vi "methane_reactor_run.vi"() -> ()   [LabVIEW 2019]
uses:
  <vilib>/Utility/sysdir.llb/System Directory Type.ctl
  lib/libSimulationControl/libSimulationControl.lvlib
  lib/libFileFunctions/libFileFunctions.lvlib
panel:
  out "working_directory_tmp":string
  out "working_directory":string
  out "time":dbl
  out "starttime":dbl
  out "standard output":string
  out "standard error":string
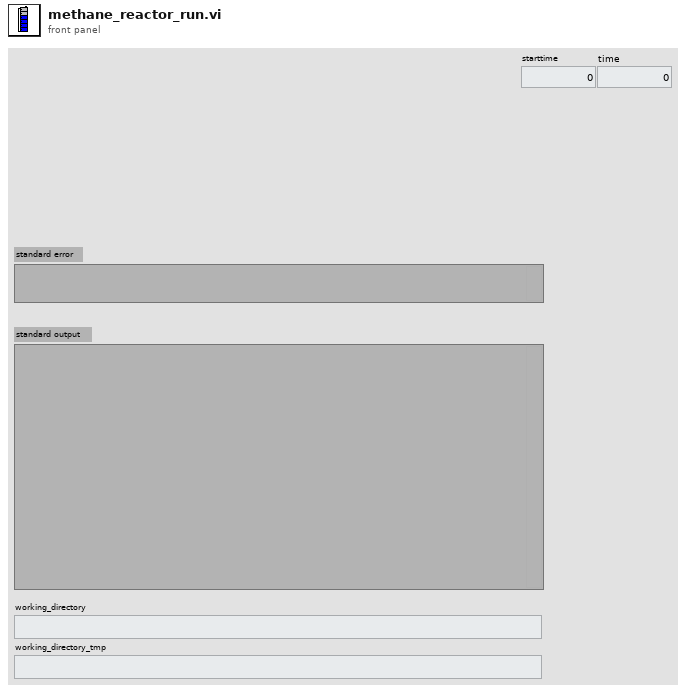
[diagram p1: front panel]
types:
  T1 = typedef "System Directory Type.ctl" = i32
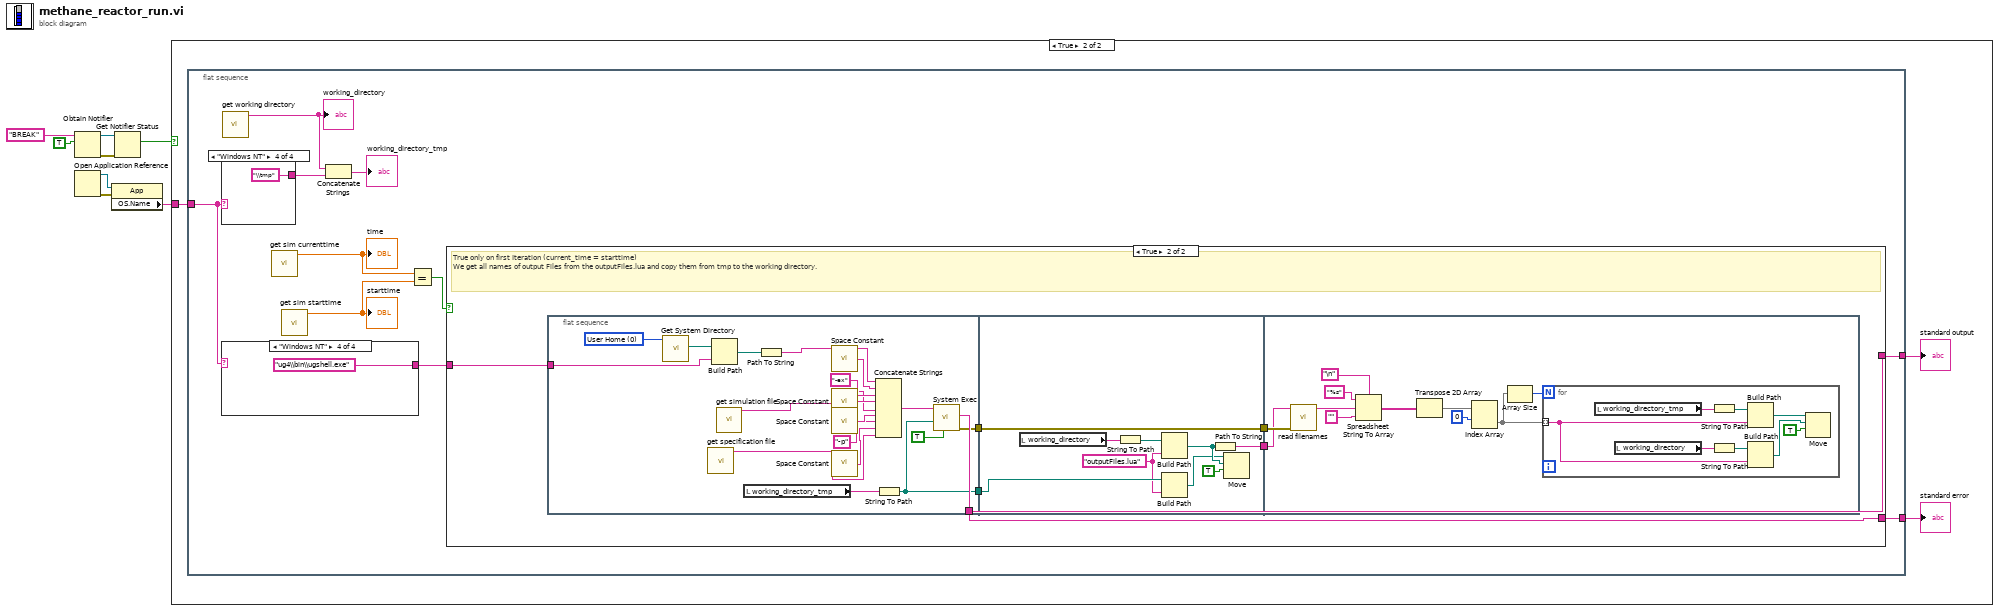
[diagram p0: block diagram]
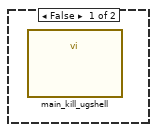
[diagram p2: hidden frame]
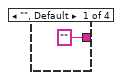
[diagram p3: hidden frame]
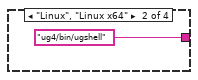
[diagram p4: hidden frame]
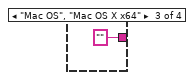
[diagram p5: hidden frame]
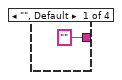
[diagram p6: hidden frame]
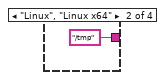
[diagram p7: hidden frame]
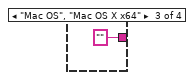
[diagram p8: hidden frame]
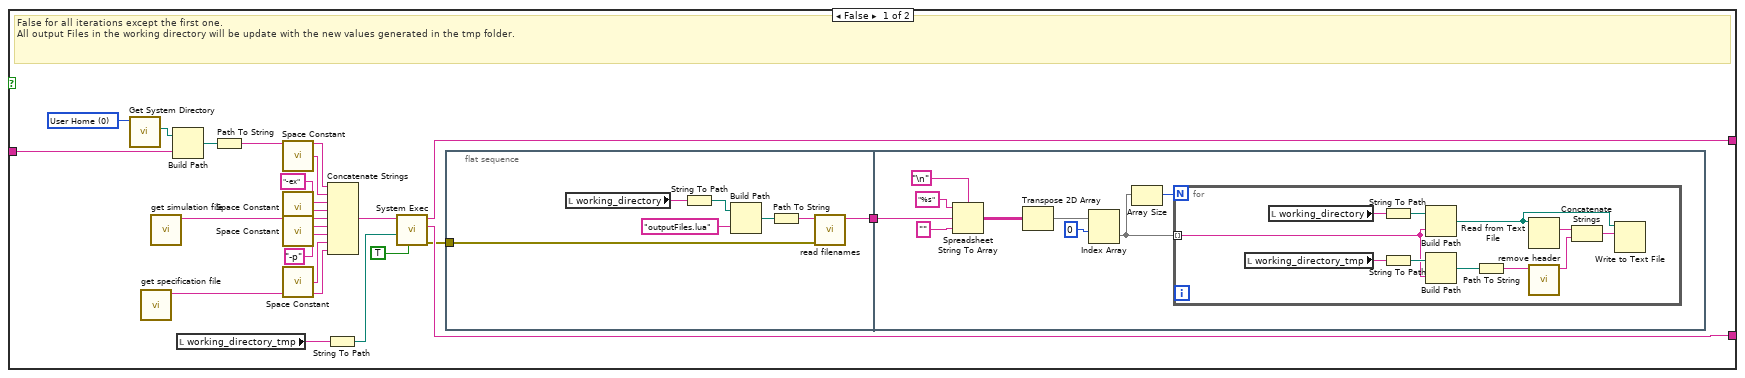
[diagram p9: hidden frame]
diagram:
  n1 = Obtain Notifier(name (unnamed)="BREAK", notification data type=TRUE) -> (notifier out=w6:refnum<notifier>, error out=w5:errorcluster)  [unwired: 2 in, 1 out]
  n2 = Open Application Reference() -> (0:w2:errorcluster, 3:w3:refnum<vi>)  [unwired: 4 in]
  n3 = property class="App"(reference=w3, error in=w2) -> ("OS.Name"=w1:string)  [unwired: 2 out]
  n4 = Get Notifier Status(notifier=w6, error in (no error)=w5) -> (current notification=w4:bool)  [unwired: 4 out]
  n5 = case shown="True" w4 {
    tunnel: w1 -> [_ w9]
    frame False {
      n6 = call "main_kill_ugshell.vi"() -> ()  [unwired: 12 in]
    }
    frame True {
      n7 = flat-sequence {
        tunnel: [w20] -> w11
        tunnel: [w19] -> w10
        tunnel: w9 -> [w13]
        frame #0 {
          n8 = case shown="\"Windows NT\"" w13 {
            tunnel: ["" ("return type") "/tmp" ("name or relative path") "" ("return type") "\\tmp" ("name or relative path")] -> w14
            frame "", Default {
            }
            frame "Linux", "Linux x64" {
            }
            frame "Mac OS", "Mac OS X x64" {
            }
            frame "Windows NT" {
            }
          }
          n9 = case shown="\"Windows NT\"" w13 {
            tunnel: ["" ("return type") "ug4/bin/ugshell" ("name or relative path") "" ("return type") "ug4\\bin\\ugshell.exe" ("name or relative path")] -> w12
            frame "", Default {
            }
            frame "Linux", "Linux x64" {
            }
            frame "Mac OS", "Mac OS X x64" {
            }
            frame "Windows NT" {
            }
          }
          n10 = call "get working directory.vi"() -> ("function return"=w15:string)  [unwired: 10 in, 1 out]
          "working_directory" <- w15
          n11 = call "get sim currenttime.vi"() -> ("function return"=w16:dbl)  [unwired: 10 in, 1 out]
          "time" <- w16
          n12 = call "get sim starttime.vi"() -> ("function return"=w17:dbl)  [unwired: 10 in, 1 out]
          "starttime" <- w17
          n13 = Concatenate Strings(w15, w14) -> (→"working_directory_tmp":string)
          n14 = Equal?(x=w16, y=w17) -> (x = y?=w21:bool)
          n15 = case shown="True" w21 {
            tunnel: [w38 w84] -> w20
            tunnel: [w37 w83] -> w19
            tunnel: w12 -> [w30 w78]
            frame False {
              w42 = T1 0 items=["User Home"=0, "User Desktop"=1, "User Documents"=2, "User Application Data"=3, "User Preferences"=4, "User Temporary"=5, "Public Documents"=6, "Public Application Data"=7, "Public Preferences"=8, "Public Cache"=13, "System Core Libraries"=9, "System Installed Libraries"=10, "Application Files"=11, "Boot Volume Root"=12] ("system directory type")
              # "False for all iterations except the first one.\nAll output Files in the working directory will be update with the new values generated in the tmp folder."
              n16 = call <vilib>:"Get System Directory.vi"("system directory type"=w42) -> ("system directory"=w49:path)  [unwired: 10 in]
              n17 = call "get specification file.vi"() -> ("function return"=w32:string)  [unwired: 10 in, 1 out]
              n18 = call "get simulation file.vi"() -> ("function return"=w33:string)  [unwired: 10 in, 1 out]
              n19 = Build Path(base path=w49, name or relative path=w30) -> (appended path=w47:path)
              n20 = local read "working_directory_tmp"() -> (w34:string)
              n21 = Path To String(path=w47) -> (string=w43:string)
              n22 = call <vilib>:"Space Constant.vi"() -> ("String"=w44:string)
              n23 = call <vilib>:"Space Constant.vi"() -> ("String"=w45:string)
              n24 = call <vilib>:"Space Constant.vi"() -> ("String"=w46:string)
              n25 = call <vilib>:"Space Constant.vi"() -> ("String"=w50:string)
              n26 = String To Path(string=w34) -> (path=w39:path)
              n27 = Concatenate Strings(w43, w44, "-ex" ("command line"), w45, w33, w46, "-p" ("command line"), w50, w32) -> (w48:string)
              n28 = call <vilib>:"System Exec.vi"("run minimized? (F)"=TRUE, "working directory"=w39, "command line"=w48) -> ("error out"=w36:errorcluster, "standard error"=w37:string, "standard output"=w38:string)  [unwired: 5 in, 1 out]
              n29 = flat-sequence {
                tunnel: w36 -> [w57]
                tunnel: [w56] -> w35
                tunnel: w35 -> [w58]
                frame #0 {
                  n30 = local read "working_directory"() -> (w54:string)
                  n31 = String To Path(string=w54) -> (path=w53:path)
                  n32 = Build Path(base path=w53, name or relative path="outputFiles.lua" ("string")) -> (appended path=w52:path)
                  n33 = Path To String(path=w52) -> (string=w51:string)
                  n34 = call "read filenames.vi"("error in (no error)"=w57, "path"=w51) -> ("function return"=w56:string)  [unwired: 8 in, 1 out]
                }
                frame #1 {
                  n35 = Spreadsheet String To Array(delimiter (Tab)="\n", format string="%s", spreadsheet string=w58, array type (2D Dbl)="") -> (array=w64:string[][])
                  n36 = Transpose 2D Array(2D array=w64) -> (transposed array=w65:string[][])
                  n37 = Index Array(array=w65, index (row)=0) -> (element=w59:string[])  [unwired: 1 in]
                  n38 = Array Size(array=w59) -> (size(s)=w66:i32)
                  n39 = for {
                    N: w66 -> [_]
                    tunnel: w59 -> [w70] mode=indexing
                    n40 = local read "working_directory_tmp"() -> (w72:string)
                    n41 = local read "working_directory"() -> (w75:string)
                    n42 = String To Path(string=w75) -> (path=w74:path)
                    n43 = String To Path(string=w72) -> (path=w71:path)
                    n44 = Build Path(base path=w74, name or relative path=w70) -> (appended path=w73:path)
                    n45 = Build Path(base path=w71, name or relative path=w70) -> (appended path=w69:path)
                    n46 = Path To String(path=w69) -> (string=w68:string)
                    n47 = Read from Text File(file (use dialog)=w73) -> (text=w77:string)  [unwired: 3 in, 3 out]
                    n48 = call "remove header.vi"("path"=w68) -> ("function return"=w67:string)  [unwired: 9 in, 1 out]
                    n49 = Concatenate Strings(w77, w67) -> (w76:string)
                    n50 = Write to Text File(file (use dialog)=w73, text=w76) -> ()  [unwired: 2 in, 3 out]
                  }
                }
              }
            }
            frame True {
              # "True only on first Iteration (current_time = starttime)\nWe get all names of output Files from the outputFiles.lua and copy them from tmp to the working directory."
              n51 = flat-sequence {
                tunnel: [w93] -> w84
                tunnel: [w92] -> w83
                tunnel: [w91] -> w81
                tunnel: [w89] -> w80
                tunnel: w78 -> [w86]
                tunnel: [w112] -> w82
                tunnel: w81 -> [w112]
                tunnel: w80 -> [w111]
                tunnel: [w107] -> w79
                tunnel: w82 -> [w116]
                tunnel: w79 -> [w115]
                frame #0 {
                  w96 = T1 0 items=["User Home"=0, "User Desktop"=1, "User Documents"=2, "User Application Data"=3, "User Preferences"=4, "User Temporary"=5, "Public Documents"=6, "Public Application Data"=7, "Public Preferences"=8, "Public Cache"=13, "System Core Libraries"=9, "System Installed Libraries"=10, "Application Files"=11, "Boot Volume Root"=12] ("system directory type")
                  n52 = call <vilib>:"Get System Directory.vi"("system directory type"=w96) -> ("system directory"=w103:path)  [unwired: 10 in]
                  n53 = call "get specification file.vi"() -> ("function return"=w87:string)  [unwired: 10 in, 1 out]
                  n54 = Build Path(base path=w103, name or relative path=w86) -> (appended path=w101:path)
                  n55 = call "get simulation file.vi"() -> ("function return"=w88:string)  [unwired: 10 in, 1 out]
                  n56 = local read "working_directory_tmp"() -> (w90:string)
                  n57 = Path To String(path=w101) -> (string=w97:string)
                  n58 = call <vilib>:"Space Constant.vi"() -> ("String"=w98:string)
                  n59 = call <vilib>:"Space Constant.vi"() -> ("String"=w99:string)
                  n60 = call <vilib>:"Space Constant.vi"() -> ("String"=w100:string)
                  n61 = call <vilib>:"Space Constant.vi"() -> ("String"=w104:string)
                  n62 = Concatenate Strings(w97, w98, "-ex" ("command line"), w99, w88, w100, "-p" ("command line"), w104, w87) -> (w102:string)
                  n63 = String To Path(string=w90) -> (path=w89:path)
                  n64 = call <vilib>:"System Exec.vi"("run minimized? (F)"=TRUE, "working directory"=w89, "command line"=w102) -> ("error out"=w91:errorcluster, "standard error"=w92:string, "standard output"=w93:string)  [unwired: 5 in, 1 out]
                }
                frame #1 {
                  w108 = "outputFiles.lua" ("string")
                  n65 = local read "working_directory"() -> (w110:string)
                  n66 = String To Path(string=w110) -> (path=w109:path)
                  n67 = Build Path(base path=w109, name or relative path=w108) -> (appended path=w106:path)
                  n68 = Build Path(base path=w111, name or relative path=w108) -> (appended path=w105:path)
                  n69 = Path To String(path=w106) -> (string=w107:string)
                  n70 = Move(source path=w105, 9:TRUE ("overwrite (F)"), 10:w106) -> ()  [unwired: 2 in, 3 out]
                }
                frame #2 {
                  n71 = call "read filenames.vi"("error in (no error)"=w116, "path"=w115) -> ("function return"=w114:string)  [unwired: 8 in, 1 out]
                  n72 = Spreadsheet String To Array(delimiter (Tab)="\n", format string="%s", spreadsheet string=w114, array type (2D Dbl)="") -> (array=w122:string[][])
                  n73 = Transpose 2D Array(2D array=w122) -> (transposed array=w123:string[][])
                  n74 = Index Array(array=w123, index (row)=0) -> (element=w117:string[])  [unwired: 1 in]
                  n75 = Array Size(array=w117) -> (size(s)=w124:i32)
                  n76 = for {
                    N: w124 -> [_]
                    tunnel: w117 -> [w128] mode=indexing
                    n77 = local read "working_directory_tmp"() -> (w130:string)
                    n78 = local read "working_directory"() -> (w127:string)
                    n79 = String To Path(string=w130) -> (path=w129:path)
                    n80 = String To Path(string=w127) -> (path=w125:path)
                    n81 = Build Path(base path=w129, name or relative path=w128) -> (appended path=w131:path)
                    n82 = Build Path(base path=w125, name or relative path=w128) -> (appended path=w126:path)
                    n83 = Move(source path=w131, 9:TRUE ("overwrite (F)"), 10:w126) -> ()  [unwired: 2 in, 3 out]
                  }
                }
              }
            }
          }
        }
      }
      "standard error" <- w10
      "standard output" <- w11
    }
  }
